vi "Build VariantToAttribute.vi"(8 "error in (no error)":errorcluster, 10 "Get Type VI":refnum<vi>, 11 "CS++Actor in":refnum<class "CS++Actor.lvclass">) -> (0 "error out":errorcluster, 3 "CS++Actor out":refnum<class "CS++Actor.lvclass">)   [LabVIEW 2016, in "CS++Actor.lvlib" / "CS++Actor.lvclass"]
uses:
  CS++Actor.lvclass
  CS++Actor.lvclass/CS++Actor.ctl
  <vilib>/Utility/traverseref.llb/TRef TravTarget.ctl
  <vilib>/Utility/miscctls.llb/LVPositionTypeDef.ctl
  <vilib>/Utility/traverseref.llb/VI Scripting - Traverse.lvlib
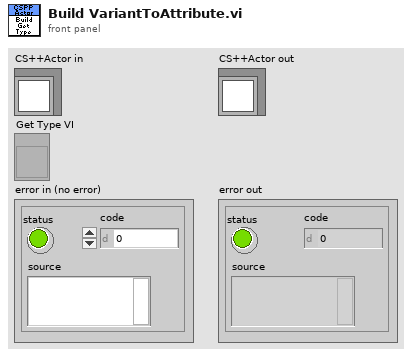
[diagram p1: front panel]
types:
  T1 = enum16{"Replace Class Controls/Indicator", "PrepareVariant2Data", "ConnectBundler"}
  T2 = enum16{"Invalid Wire Rule", "Required", "Recommended", "Optional", "Dynamic Dispatch"}
  T3 = typedef "TRef TravTarget.ctl" = enum16{"FP", "BD", "Other"}
  T4 = typedef "LVPositionTypeDef.ctl" = cluster{"Left":i32, "Top":i32}
  T5 = typedef "LVRectTypeDef.ctl" = cluster{"Left":i16, "Top":i16, "Right":i16, "Bottom":i16}
  T6 = enum16{"Invalid Wire Rule", "Required", "Recommended", "Optional", "Dynamic Dispatch"}[]
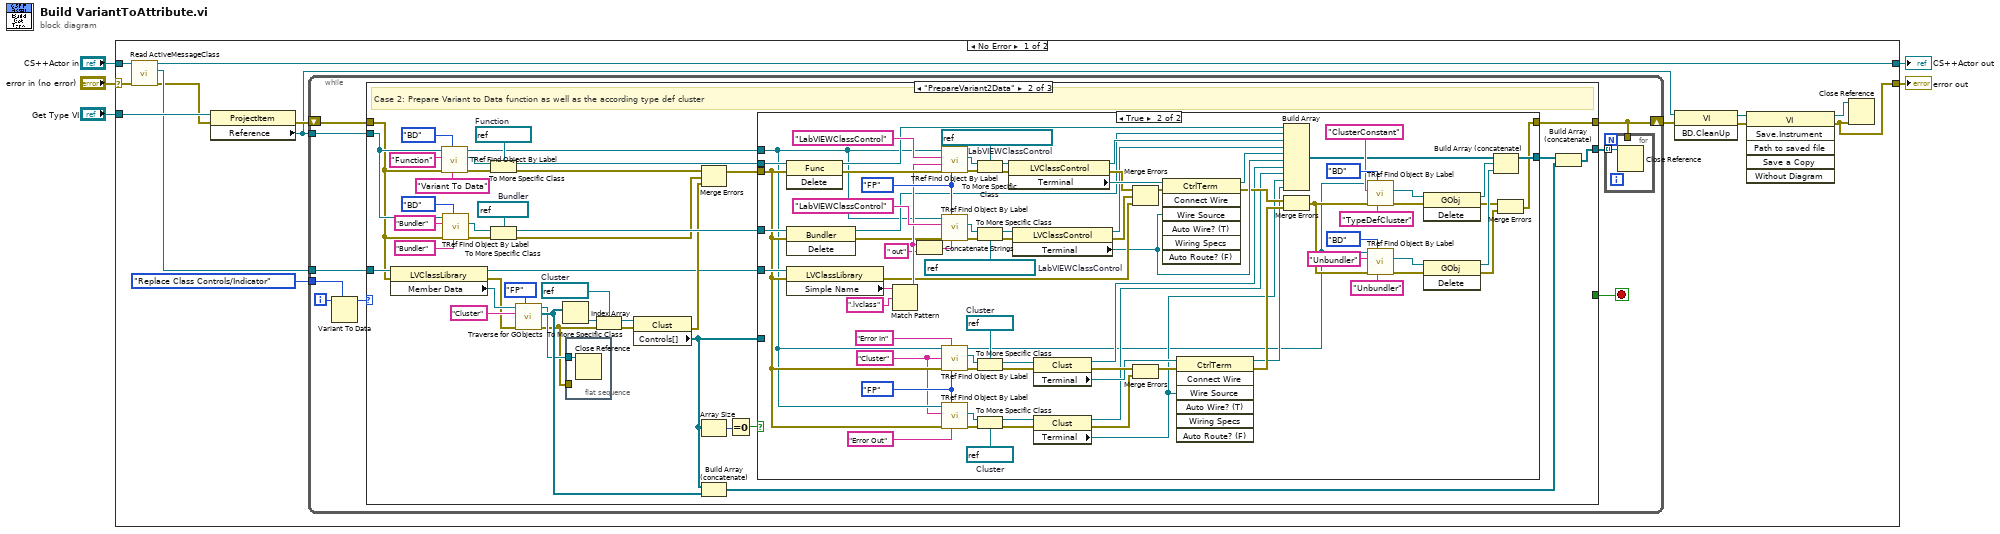
[diagram p0: block diagram]
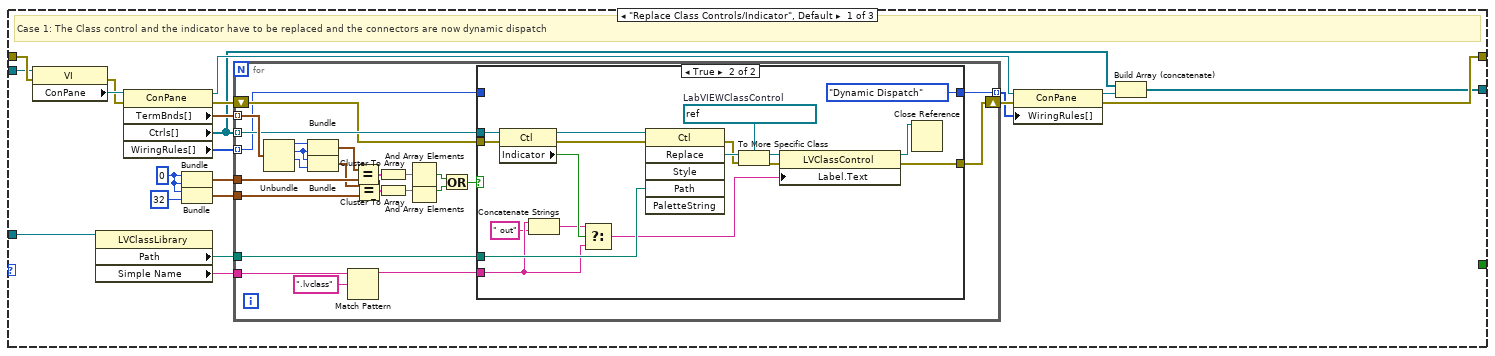
[diagram p2: hidden frame]
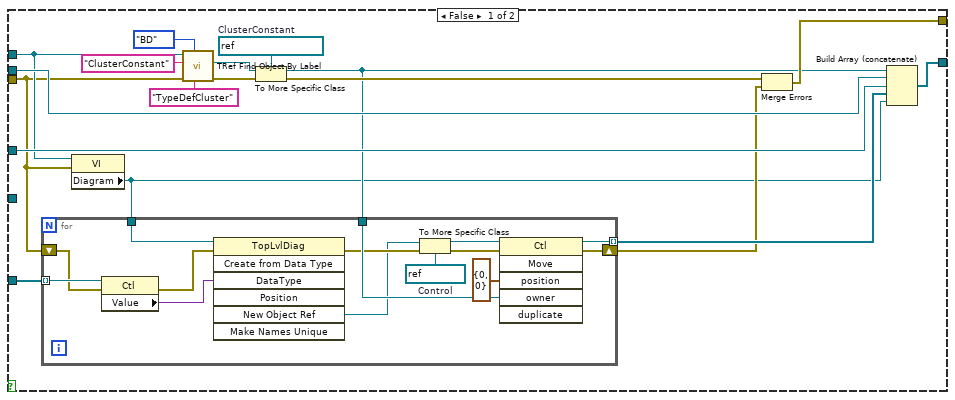
[diagram p4: hidden frame]
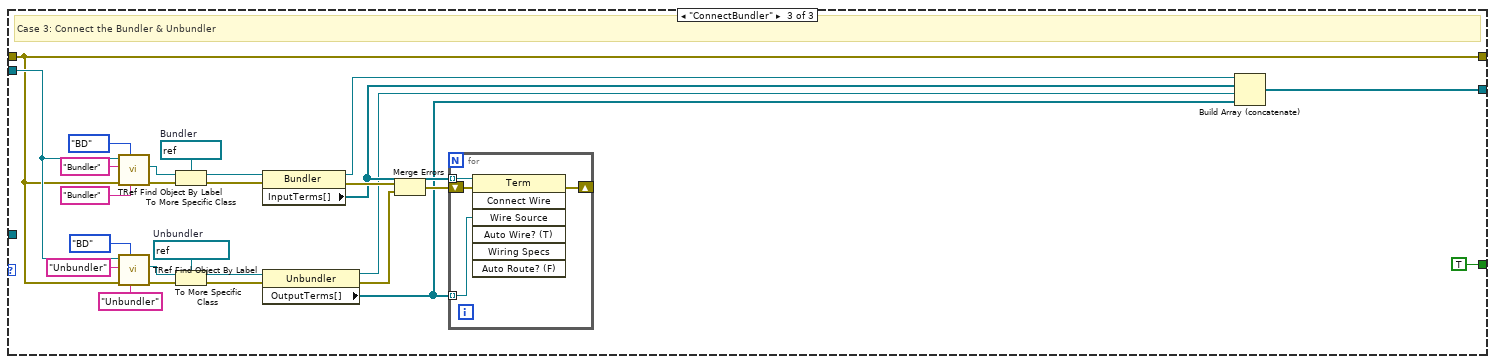
[diagram p5: hidden frame]
diagram:
  n1 = case shown="No Error" "error in (no error)" {
    selector: "error in (no error)" -> [w6 w280]
    tunnel: [w12 w280] -> w4
    tunnel: [w8 w279] -> w2
    tunnel: "CS++Actor in" -> [w7 w279]
    tunnel: "Get Type VI" -> [w18 _]
    frame No Error {
      n2 = call "Read ActiveMessageClass.vi"("error in (no error)"=w6, "CS++Actor in"=w7) -> ("error out"=w9:errorcluster, "ActiveMessageClass"=w10:refnum<vi>, "CS++Actor out"=w8:refnum<class "CS++Actor.lvclass">)  [unwired: 7 in]
      n3 = property class="ProjectItem"(reference=w18, error in=w9) -> (error out=w17:errorcluster, "Reference"=w13:refnum<vi>)  [unwired: 1 out]
      n4 = while {
        tunnel: T1."Replace Class Controls/Indicator" -> [w27]
        tunnel: w13 -> [w24]
        shift-right: [w20] -> w11
        shift-left: w17 -> [w25]
        tunnel: w10 -> [w23]
        i -> [w28]
        stop <- w22 stop-if-true
        n5 = Variant To Data(type=w27, Variant=w28) -> (data=w26:T1)  [unwired: 1 in, 1 out]
        n6 = case shown="\"PrepareVariant2Data\"" w26 {
          tunnel: w25 -> [w33 w106 w259]
          tunnel: w24 -> [w32 w107 w260]
          tunnel: w23 -> [w31 w121 _]
          tunnel: [w30 w101 w259] -> w20
          tunnel: [_ _ TRUE] -> w22
          tunnel: [w29 w98 w247] -> w21
          frame "Replace Class Controls/Indicator", Default {
            w41 = i16 0
            # "Case 1: The Class control and the indicator have to be replaced and the connectors are now dynamic dispatch"
            n7 = property class="VI"(reference=w32, error in=w33) -> (error out=w48:errorcluster, "ConPane"=w49:refnum<vi>)  [unwired: 1 out]
            n8 = property class="LVClassLibrary"(reference=w31) -> ("Path"=w42:path, "Simple Name"=w34:string)  [unwired: 1 in, 2 out]
            n9 = property class="ConPane"(reference=w49, error in=w48) -> (reference out=w38:refnum<vi>, error out=w46:errorcluster, "TermBnds[]"=w47:T5[], "Ctrls[]"=w36:refnum<vi>[], "WiringRules[]"=w40:T6)
            n10 = Bundle(w41, w41) -> (w44:cluster{i16, i16})  [unwired: 1 in]
            n11 = Bundle(w41, i16 32) -> (w43:cluster{i16, i16})  [unwired: 1 in]
            n12 = for {
              tunnel: w47 -> [w73] mode=indexing
              tunnel: w36 -> [w63] mode=indexing
              shift-right: [w57] -> w39
              shift-left: w46 -> [w62]
              tunnel: w44 -> [w70]
              tunnel: w43 -> [w68]
              tunnel: w42 -> [w58]
              tunnel: w40 -> [w54] mode=indexing
              tunnel: [w53] -> w37 mode=indexing
              tunnel: w34 -> [w52]
              n13 = Unbundle(w73) -> ("Left"=w72:i16, "Top"=w55:i16, "Right"=w56:i16)  [unwired: 1 out]
              n14 = Bundle("Left"=w72, "Top"=w55) -> (w71:cluster{"Left":i16, "Top":i16})  [unwired: 1 in]
              n15 = Bundle("Top"=w55, "Right"=w56) -> (w69:cluster{"Top":i16, "Right":i16})  [unwired: 1 in]
              n16 = Match Pattern(string=w52, regular expression=".lvclass") -> (before substring=w51:string)  [unwired: 1 in, 3 out]
              n17 = Equal?(x=w71, y=w70) -> (x = y?=w67:cluster{bool, bool})
              n18 = Equal?(x=w69, y=w68) -> (x = y?=w66:cluster{bool, bool})
              n19 = Cluster To Array(cluster=w67) -> (array=w65:bool[])
              n20 = Cluster To Array(cluster=w66) -> (array=w64:bool[])
              n21 = And Array Elements(Boolean array=w65) -> (logical AND=w61:bool)
              n22 = And Array Elements(Boolean array=w64) -> (logical AND=w60:bool)
              n23 = Or(x=w61, y=w60) -> (x .or. y?=w59:bool)
              n24 = case shown="True" w59 {
                tunnel: w63 -> [_ w84]
                tunnel: w62 -> [w75 w83]
                tunnel: [w75 w86] -> w57
                tunnel: w58 -> [_ w93]
                tunnel: w54 -> [w74 _]
                tunnel: [w74 T2."Dynamic Dispatch" ("Wire Rule")] -> w53
                tunnel: w51 -> [_ w78]
                frame False {
                }
                frame True {
                  w91 = refnum<vi> refnum  # LabVIEWClassControl
                  n25 = property class="Ctl"(reference=w84, error in=w83) -> (reference out=w81:refnum<vi>, error out=w82:errorcluster, "Indicator"=w80:bool)
                  n26 = Concatenate Strings(w78, " out" ("string")) -> (w77:string)
                  n27 = Select(t=w77, s=w80, f=w78) -> (s? t:f=w79:string)
                  n28 = invoke class="Ctl" method="Replace"(reference=w81, error in=w82, "Path"=w93) -> (error out=w87:errorcluster, "Replace"=w90:refnum<vi>)  [unwired: 3 in, 4 out]
                  n29 = To More Specific Class(target class=w91, reference=w90, error in=w87) -> (specific class reference=w89:refnum<vi>, error out=w88:errorcluster)
                  n30 = property class="LVClassControl"(reference=w89, error in=w88, "Label.Text"=w79) -> (reference out=w85:refnum<vi>, error out=w86:errorcluster)
                  n31 = Close Reference(reference=w85) -> ()  [unwired: 1 in, 1 out]
                }
              }
            }
            n32 = property class="ConPane"(reference=w38, error in=w39, "WiringRules[]"=w37) -> (reference out=w35:refnum<vi>, error out=w30:errorcluster)
            n33 = Build Array (concatenate)(w36, w35) -> (w29:refnum<vi>[])
          }
          frame "PrepareVariant2Data" {
            w108 = refnum<vi> refnum  # Bundler
            w125 = refnum<vi> refnum  # Cluster
            w133 = refnum<vi> refnum  # Function
            # "Case 2: Prepare Variant to Data function as well as the according type def cluster"
            n34 = property class="LVClassLibrary"(reference=w121, error in=w106) -> (reference out=w102:refnum<vi>, error out=w120:errorcluster, "Member Data"=w122:refnum<vi>)
            n35 = call <vilib>:"TRef Find Object By Label.vi"("Label"="Variant To Data", "Traverse Target"=TRef_TravTarget."BD", "error in (no error)"=w106, "Class Name"="Function", "VI Ref"=w107) -> ("error out"=w132:errorcluster, "Found Obj Ref"=w131:refnum<vi>, "dup VI Ref"=w114:refnum<vi>)  [unwired: 3 in, 1 out]
            n36 = call <vilib>:"TRef Find Object By Label.vi"("Label"="Bundler", "Traverse Target"=TRef_TravTarget."BD", "error in (no error)"=w106, "Class Name"="Bundler", "VI Ref"=w107) -> ("error out"=w110:errorcluster, "Found Obj Ref"=w109:refnum<vi>)  [unwired: 3 in, 2 out]
            n37 = To More Specific Class(target class=w133, reference=w131, error in=w132) -> (specific class reference=w117:refnum<vi>, error out=w116:errorcluster)
            n38 = To More Specific Class(target class=w108, reference=w109, error in=w110) -> (specific class reference=w105:refnum<vi>, error out=w103:errorcluster)
            n39 = call <vilib>:"Traverse for GObjects.vi"("Traverse Target"=TRef_TravTarget."FP", "error in (no error)"=w120, "Class Name"="Cluster" ("name/order"), "VI Refnum"=w122) -> ("error out"=w94:errorcluster, "References"=w100:refnum<vi>[], "dup VI Refnum"=w95:refnum<vi>)  [unwired: 4 in, 1 out]
            n40 = Index Array(array=w100) -> (element=w126:refnum<vi>)  [unwired: 1 in]
            n41 = flat-sequence {
              tunnel: w95 -> [w135]
              tunnel: w94 -> [_]
              frame #0 {
                n42 = Close Reference(reference=w135) -> ()  [unwired: 1 in, 1 out]
              }
            }
            n43 = To More Specific Class(target class=w125, reference=w126, error in=w94) -> (specific class reference=w123:refnum<vi>, error out=w124:errorcluster)
            n44 = property class="Clust"(reference=w123, error in=w124) -> (error out=w104:errorcluster, "Controls[]"=w99:refnum<vi>[])  [unwired: 1 out]
            n45 = Merge Errors(w116, w103, w104) -> (w115:errorcluster)
            n46 = Array Size(array=w99) -> (size(s)=w119:i32)
            n47 = Build Array (concatenate)(w99, w100) -> (w97:refnum<vi>[])
            n48 = Equal To 0?(x=w119) -> (x = 0?=w118:bool)
            n49 = case shown="True" w118 {
              tunnel: w117 -> [w145 w245]
              tunnel: w115 -> [w136 w211]
              tunnel: w114 -> [w138 w210]
              tunnel: w105 -> [w146 w246]
              tunnel: w99 -> [w147 _]
              tunnel: w102 -> [_ w243]
              tunnel: [w142 w169] -> w101
              tunnel: [w143 w179] -> w96
              frame False {
                w150 = refnum<vi> refnum  # ClusterConstant
                n50 = property class="VI"(reference=w138, error in=w136) -> ("Diagram"=w137:refnum<vi>)  [unwired: 2 out]
                n51 = call <vilib>:"TRef Find Object By Label.vi"("Label"="TypeDefCluster", "Traverse Target"=TRef_TravTarget."BD", "error in (no error)"=w136, "Class Name"="ClusterConstant", "VI Ref"=w138) -> ("error out"=w149:errorcluster, "Found Obj Ref"=w148:refnum<vi>)  [unwired: 3 in, 2 out]
                n52 = To More Specific Class(target class=w150, reference=w148, error in=w149) -> (specific class reference=w139:refnum<vi>, error out=w141:errorcluster)
                n53 = for {
                  tunnel: w147 -> [w163] mode=indexing
                  tunnel: [w167] -> w144 mode=indexing
                  shift-right: [w166] -> w140
                  shift-left: w136 -> [w162]
                  tunnel: w139 -> [w165]
                  tunnel: w137 -> [w157]
                  w159 = refnum<vi> refnum  # Control
                  n54 = property class="Ctl"(reference=w163, error in=w162) -> (error out=w161:errorcluster, "Value"=w160:variant)  [unwired: 1 out]
                  n55 = invoke class="TopLvlDiag" method="Create from Data Type"(reference=w157, error in=w161, "DataType"=w160) -> (error out=w158:errorcluster, "New Object Ref"=w156:refnum<vi>)  [unwired: 4 in, 5 out]
                  n56 = To More Specific Class(target class=w159, reference=w156, error in=w158) -> (specific class reference=w155:refnum<vi>, error out=w154:errorcluster)
                  n57 = invoke class="Ctl" method="Move"(reference=w155, error in=w154, "position"=T4 {"Left"=0, "Top"=0}, "owner"=w165) -> (reference out=w167:refnum<vi>, error out=w166:errorcluster)  [unwired: 2 in, 4 out]
                }
                n58 = Merge Errors(w141, w140) -> (w142:errorcluster)
                n59 = Build Array (concatenate)(w139, w145, w146, w144, w137) -> (w143:refnum<vi>[])
              }
              frame True {
                w202 = refnum<vi> refnum  # Cluster
                w203 = refnum<vi> refnum  # Cluster
                w197 = "Cluster" ("string")
                w212 = TRef_TravTarget."FP" ("Traverse Target")
                w232 = refnum<vi> refnum  # LabVIEWClassControl
                w231 = refnum<vi> refnum  # LabVIEWClassControl
                w238 = TRef_TravTarget."FP" ("Traverse Target")
                n60 = invoke class="Func" method="Delete"(reference=w245, error in=w211) -> (reference out=w215:refnum<vi>, error out=w241:errorcluster)  [unwired: 1 in, 1 out]
                n61 = invoke class="Bundler" method="Delete"(reference=w246, error in=w211) -> (reference out=w216:refnum<vi>, error out=w230:errorcluster)  [unwired: 1 in, 1 out]
                n62 = property class="LVClassLibrary"(reference=w243, error in=w211) -> (error out=w221:errorcluster, "Simple Name"=w242:string)  [unwired: 1 out]
                n63 = Match Pattern(string=w242, regular expression=".lvclass") -> (before substring=w237:string)  [unwired: 1 in, 3 out]
                n64 = Concatenate Strings(w237, " out" ("string")) -> (w214:string)
                n65 = call <vilib>:"TRef Find Object By Label.vi"("Label"=w237, "Traverse Target"=w238, "error in (no error)"=w241, "Class Name"="LabVIEWClassControl", "VI Ref"=w210) -> ("error out"=w235:errorcluster, "Found Obj Ref"=w236:refnum<vi>)  [unwired: 3 in, 2 out]
                n66 = call <vilib>:"TRef Find Object By Label.vi"("Label"=w214, "Traverse Target"=w238, "error in (no error)"=w230, "Class Name"="LabVIEWClassControl", "VI Ref"=w210) -> ("error out"=w234:errorcluster, "Found Obj Ref"=w233:refnum<vi>)  [unwired: 3 in, 2 out]
                n67 = call <vilib>:"TRef Find Object By Label.vi"("Label"="Error In" ("string"), "Traverse Target"=w212, "error in (no error)"=w211, "Class Name"=w197, "VI Ref"=w210) -> ("error out"=w207:errorcluster, "Found Obj Ref"=w205:refnum<vi>, "dup VI Ref"=w172:refnum<vi>)  [unwired: 3 in, 1 out]
                n68 = call <vilib>:"TRef Find Object By Label.vi"("Label"="Error Out" ("string"), "Traverse Target"=w212, "error in (no error)"=w211, "Class Name"=w197, "VI Ref"=w210) -> ("error out"=w206:errorcluster, "Found Obj Ref"=w204:refnum<vi>)  [unwired: 3 in, 2 out]
                n69 = To More Specific Class(target class=w231, reference=w236, error in=w235) -> (specific class reference=w229:refnum<vi>, error out=w228:errorcluster)
                n70 = To More Specific Class(target class=w232, reference=w233, error in=w234) -> (specific class reference=w227:refnum<vi>, error out=w226:errorcluster)
                n71 = To More Specific Class(target class=w203, reference=w205, error in=w207) -> (specific class reference=w201:refnum<vi>, error out=w200:errorcluster)
                n72 = To More Specific Class(target class=w202, reference=w204, error in=w206) -> (specific class reference=w198:refnum<vi>, error out=w199:errorcluster)
                n73 = property class="LVClassControl"(reference=w229, error in=w228) -> (reference out=w217:refnum<vi>, error out=w224:errorcluster, "Terminal"=w225:refnum<vi>)
                n74 = property class="LVClassControl"(reference=w227, error in=w226) -> (reference out=w218:refnum<vi>, error out=w222:errorcluster, "Terminal"=w219:refnum<vi>)
                n75 = property class="Clust"(reference=w201, error in=w200) -> (reference out=w190:refnum<vi>, error out=w196:errorcluster, "Terminal"=w193:refnum<vi>)
                n76 = property class="Clust"(reference=w198, error in=w199) -> (reference out=w189:refnum<vi>, error out=w195:errorcluster, "Terminal"=w187:refnum<vi>)
                n77 = Merge Errors(w224, w222, w221) -> (w223:errorcluster)
                n78 = Merge Errors(w196, w195) -> (w194:errorcluster)
                n79 = invoke class="CtrlTerm" method="Connect Wire"(reference=w225, error in=w223, "Wire Source"=w219) -> (reference out=w220:refnum<vi>, error out=w191:errorcluster)  [unwired: 4 in, 5 out]
                n80 = invoke class="CtrlTerm" method="Connect Wire"(reference=w193, error in=w194, "Wire Source"=w187) -> (reference out=w188:refnum<vi>, error out=w192:errorcluster)  [unwired: 4 in, 5 out]
                n81 = Build Array(w215, w216, w217, w218, w220, w219, w190, w189, w187, w188) -> (w180:refnum<vi>[])
                n82 = Merge Errors(w191, w192) -> (w173:errorcluster)
                n83 = call <vilib>:"TRef Find Object By Label.vi"("Label"="TypeDefCluster", "Traverse Target"=TRef_TravTarget."BD", "error in (no error)"=w173, "Class Name"="ClusterConstant", "VI Ref"=w172) -> ("error out"=w183:errorcluster, "Found Obj Ref"=w182:refnum<vi>)  [unwired: 3 in, 2 out]
                n84 = call <vilib>:"TRef Find Object By Label.vi"("Label"="Unbundler", "Traverse Target"=TRef_TravTarget."BD", "error in (no error)"=w173, "Class Name"="Unbundler", "VI Ref"=w172) -> ("error out"=w177:errorcluster, "Found Obj Ref"=w178:refnum<vi>)  [unwired: 3 in, 2 out]
                n85 = invoke class="GObj" method="Delete"(reference=w182, error in=w183) -> (reference out=w181:refnum<vi>, error out=w170:errorcluster)  [unwired: 1 in, 1 out]
                n86 = invoke class="GObj" method="Delete"(reference=w178, error in=w177) -> (reference out=w171:refnum<vi>, error out=w168:errorcluster)  [unwired: 1 in, 1 out]
                n87 = Build Array (concatenate)(w180, w181, w171) -> (w179:refnum<vi>[])
                n88 = Merge Errors(w170, w168) -> (w169:errorcluster)
              }
            }
            n89 = Build Array (concatenate)(w96, w97) -> (w98:refnum<vi>[])
          }
          frame "ConnectBundler" {
            w263 = refnum<vi> refnum  # Unbundler
            w267 = refnum<vi> refnum  # Bundler
            # "Case 3: Connect the Bundler & Unbundler"
            n90 = call <vilib>:"TRef Find Object By Label.vi"("Label"="Bundler", "Traverse Target"=TRef_TravTarget."BD", "error in (no error)"=w259, "Class Name"="Bundler", "VI Ref"=w260) -> ("error out"=w269:errorcluster, "Found Obj Ref"=w268:refnum<vi>)  [unwired: 3 in, 2 out]
            n91 = call <vilib>:"TRef Find Object By Label.vi"("Label"="Unbundler", "Traverse Target"=TRef_TravTarget."BD", "error in (no error)"=w259, "Class Name"="Unbundler", "VI Ref"=w260) -> ("error out"=w262:errorcluster, "Found Obj Ref"=w261:refnum<vi>)  [unwired: 3 in, 2 out]
            n92 = To More Specific Class(target class=w267, reference=w268, error in=w269) -> (specific class reference=w258:refnum<vi>, error out=w257:errorcluster)
            n93 = To More Specific Class(target class=w263, reference=w261, error in=w262) -> (specific class reference=w256:refnum<vi>, error out=w255:errorcluster)
            n94 = property class="Bundler"(reference=w258, error in=w257) -> (reference out=w251:refnum<vi>, error out=w254:errorcluster, "InputTerms[]"=w250:refnum<vi>[])
            n95 = property class="Unbundler"(reference=w256, error in=w255) -> (reference out=w249:refnum<vi>, error out=w253:errorcluster, "OutputTerms[]"=w248:refnum<vi>[])
            n96 = Merge Errors(w254, w253) -> (w252:errorcluster)
            n97 = for {
              shift-right: [w276] -> _
              shift-left: w252 -> [w277]
              tunnel: w250 -> [w275] mode=indexing
              tunnel: w248 -> [w274] mode=indexing
              n98 = invoke class="Term" method="Connect Wire"(reference=w275, error in=w277, "Wire Source"=w274) -> (error out=w276:errorcluster)  [unwired: 4 in, 6 out]
            }
            n99 = Build Array (concatenate)(w251, w250, w249, w248) -> (w247:refnum<vi>[])
          }
        }
        n100 = for {
          tunnel: w21 -> [w278] mode=indexing
          tunnel: w20 -> [_]
          n101 = Close Reference(reference=w278) -> ()  [unwired: 1 in, 1 out]
        }
      }
      n102 = invoke class="VI" method="BD.CleanUp"(reference=w13, error in=w11) -> (reference out=w16:refnum<vi>, error out=w14:errorcluster)  [unwired: 1 in, 1 out]
      n103 = invoke class="VI" method="Save.Instrument"(reference=w16, error in=w14) -> (reference out=w15:refnum<vi>, error out=w12:errorcluster)  [unwired: 4 in, 4 out]
      n104 = Close Reference(reference=w15, error in (no error)=w12) -> ()  [unwired: 1 out]
    }
    frame Error {
    }
  }
  "error out" <- w4
  "CS++Actor out" <- w2
